vi "SendCommand.vi"(8 "error in (no error)":errorcluster, 10 "command":string, 11 "VISA Refnum in":refnum<visa-resource-name>) -> (0 "error out":errorcluster, 2 "result":string, 3 "VISA resource name out":refnum<visa-resource-name>)   [LabVIEW 2014]
uses:
  <vilib>/Utility/error.llb/whitespace.ctl
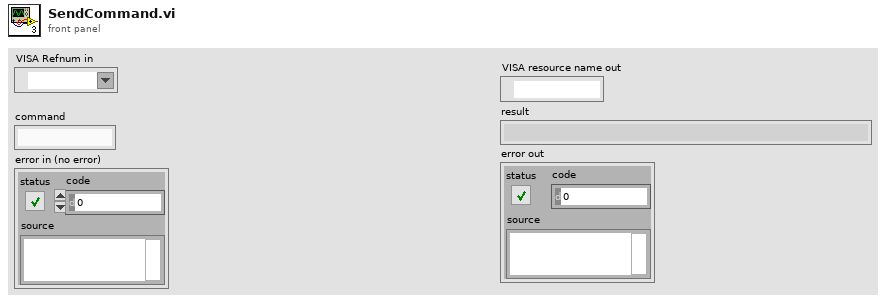
[diagram p1: front panel]
types:
  T1 = typedef "whitespace.ctl" = u16
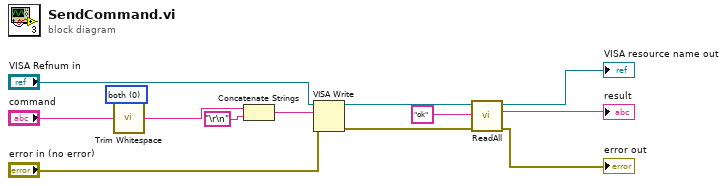
[diagram p0: block diagram]
diagram:
  w1 = T1 0 items=["both", "start of string", "end of string"] ("location (both)")
  n1 = call <vilib>:"Trim Whitespace.vi"("string"="command", "location (both)"=w1) -> ("trimmed string"=w2:string)
  n2 = Concatenate Strings(w2, "\r\n") -> (w12:string)
  n3 = VISA Write(VISA resource name="VISA Refnum in", write buffer=w12, error in (no error)="error in (no error)") -> (VISA resource name out=w10:refnum<visa-resource-name>, error out=w7:errorcluster)  [unwired: 1 out]
  n4 = call "ReadAll.vi"("error in (no error)"=w7, "value"="ok", "VISA resource in"=w10) -> ("error out"=→"error out":errorcluster, "result"=→"result":string, "VISA resource out"=→"VISA resource name out":refnum<visa-resource-name>)  [unwired: 5 in, 1 out]
